vi "APS get field bus slave first axisno.vi"(6 "TotalAxes":i32, 7 "AxisNo":i32, 8 "error in (no error)":errorcluster caption="错误输入（无错误）", 9 "MOD_No":i32, 10 "BUS_No":i32, 11 "Board_ID":i32) -> (0 "error out":errorcluster caption="错误输出", 3 "function return":i32, 4 "TotalAxes out":i32, 5 "AxisNo out":i32)   [LabVIEW 2011, in "APS168.lvlib"]
doc: "I32 FNTYPE APS_get_field_bus_slave_serialID( I32 Board_ID, I32 BUS_No, I32 MOD_No, I16 *Serial_ID ); I32 FNTYPE APS_get_field_bus_slave_first_axisno( I32 Board_ID, I32 BUS_No, I32 MOD_No, I32 *AxisNo, I32 *TotalAxes );"
uses:
  APS168.lvlib
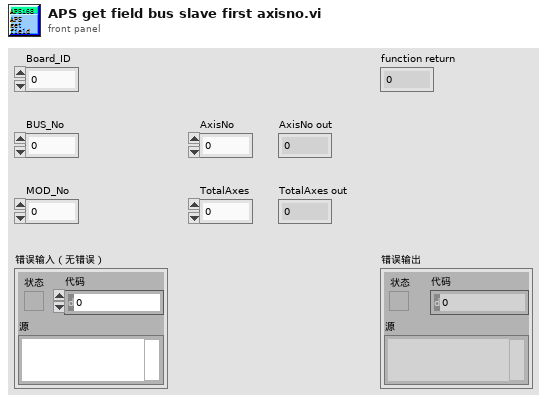
[diagram p1: front panel]
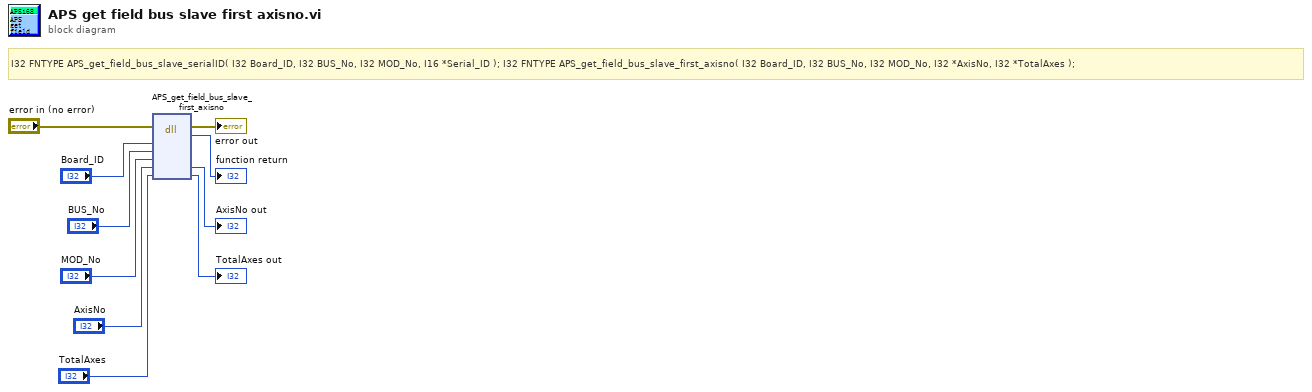
[diagram p0: block diagram]
diagram:
  # "I32 FNTYPE APS_get_field_bus_slave_serialID( I32 Board_ID, I32 BUS_No, I32 MOD_No, I16 *Serial_ID );\tI32 FNTYPE APS_get_field_bus_slave_first_axisno( I32 Board_ID, I32 BUS_No, I32 MOD_No, I32 *AxisNo, I32 *TotalAxes );"
  n1 = dll-call lib="PTH1Labs E软件ADLINK 204CAPS_1_7_1_LIB line 连续运动204APS168.*" fn="APS_get_field_bus_slave_first_axisno"(error in="error in (no error)", "Board_ID"="Board_ID", "BUS_No"="BUS_No", "MOD_No"="MOD_No", "AxisNo"="AxisNo", "TotalAxes"="TotalAxes") -> (error out=→"error out":errorcluster, →"function return":i32, "AxisNo"=→"AxisNo out":i32, "TotalAxes"=→"TotalAxes out":i32)  [unwired: 5 in, 1 out]
